vi "Read configuration.vi"(8 "error in":errorcluster, 11 "Add Module editor node in":refnum<class "Add Module editor node.lvclass">) -> (0 "error out":errorcluster, 2 "configuration":refnum<class "NISE_CEF_serializable configuration.lvclass">, 3 "Add Module editor node out":refnum<class "Add Module editor node.lvclass">)   [LabVIEW 2018, in "Add Module editor node.lvclass"]
uses:
  Add Module editor node.lvclass
  <vilib>/NI/Configuration Framework/serializable configuration/NISE_CEF_serializable configuration.lvclass
  Add Module editor node.lvclass/Add Module editor node.ctl
  module/configuration/Add Module configuration.lvclass
  C:/Program Files (x86)/National Instruments/LabVIEW 2018/vi.lib/NI/Configuration Framework/serializable configuration/NISE_CEF_serializable configuration.lvclass
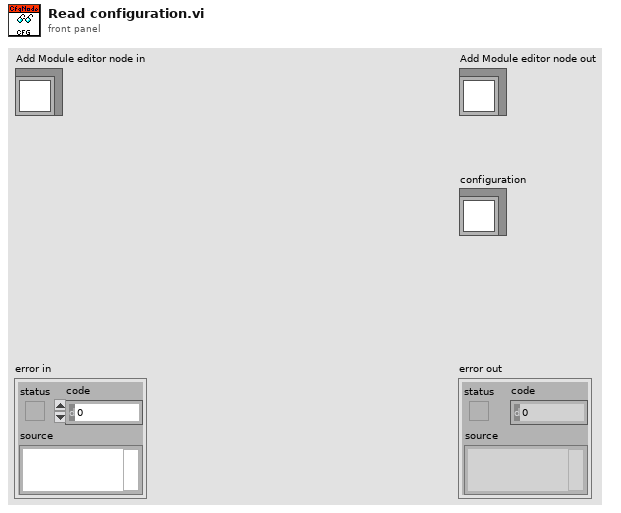
[diagram p1: front panel]
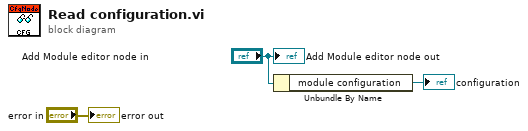
[diagram p0: block diagram]
diagram:
  n1 = Unbundle By Name("Add Module editor node in") -> ("module configuration"=→"configuration":refnum<class "Add Module configuration.lvclass">)
  "error out" <- "error in"
  "Add Module editor node out" <- "Add Module editor node in"
